vi "write_singleFIFO.vi"(10 "maximum bit depth":i8, 11 "values to be written":T1) -> (0 "FIFO overflow":bool)   [LabVIEW 2010]
uses:
  common_typedefs/channels_cluster.ctl
  <vilib>/rvi/DataTransferAndStorage/Container/XNode/niFpgaContainer.xnode
  <vilib>/rvi/DataTransferAndStorage/Container/Common/niFpgaContainerMethod.ctl
  <vilib>/rvi/DataTransferAndStorage/Container/Common/niFpgaTransferTypeControl.ctl
  <vilib>/rvi/interface/RandomDataEmulation/nirviRandomDataFPGAFIFO.vi
  <vilib>/rvi/interface/RandomDataEmulation/niFpgaRandomDataHandleErrors.vi
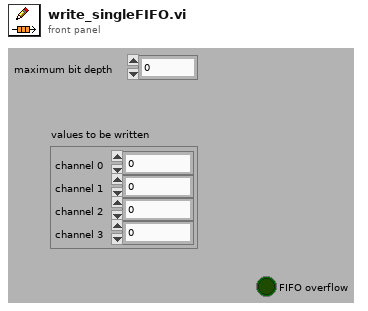
[diagram p1: front panel]
types:
  T1 = typedef "channels_cluster.ctl" = cluster{"channel 0":u32, "channel 1":u32, "channel 2":u32, "channel 3":u32}
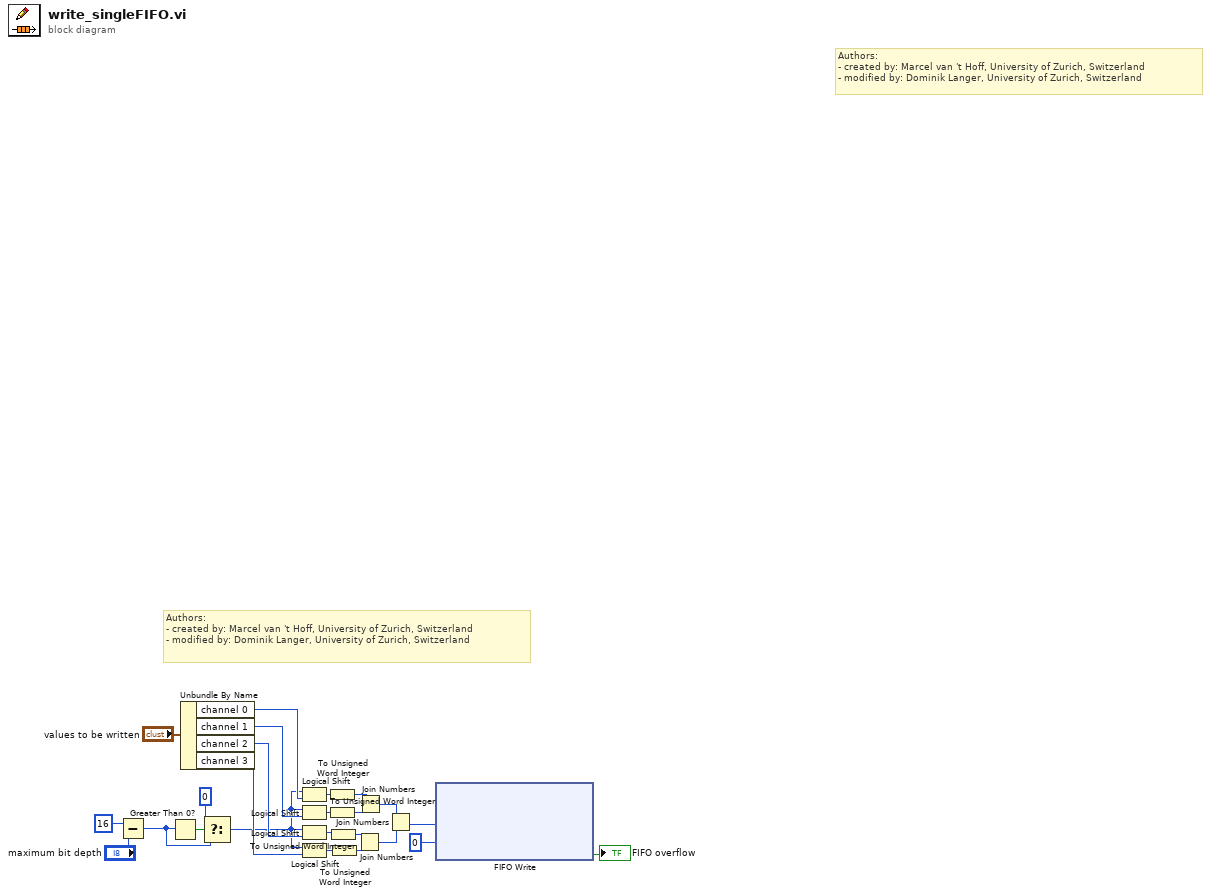
[diagram p0: block diagram]
diagram:
  # "Authors: \n- created by: Marcel van 't Hoff, University of Zurich, Switzerland\n- modified by: Dominik Langer, University of Zurich, Switzerland"
  # "Authors: \n- created by: Marcel van 't Hoff, University of Zurich, Switzerland\n- modified by: Dominik Langer, University of Zurich, Switzerland"
  n1 = Subtract(x=i8 16, y="maximum bit depth") -> (x-y=w20:i8)
  n2 = Greater Than 0?(x=w20) -> (x > 0?=w19:bool)
  n3 = Unbundle By Name("values to be written") -> ("channel 0"=w17:u32, "channel 1"=w18:u32, "channel 2"=w16:u32, "channel 3"=w13:u32)
  n4 = Select(t=i8 0 ("f"), s=w19, f=w20) -> (s? t:f=w12:i8)
  n5 = Logical Shift(y=w12, x=w17) -> (x << y=w8:u32)
  n6 = Logical Shift(y=w12, x=w18) -> (x << y=w6:u32)
  n7 = Logical Shift(y=w12, x=w16) -> (x << y=w3:u32)
  n8 = Logical Shift(y=w12, x=w13) -> (x << y=w5:u32)
  n9 = To Unsigned Word Integer(number=w8) -> (unsigned 16bit integer=w7:u16)
  n10 = To Unsigned Word Integer(number=w6) -> (unsigned 16bit integer=w1:u16)
  n11 = To Unsigned Word Integer(number=w3) -> (unsigned 16bit integer=w2:u16)
  n12 = To Unsigned Word Integer(number=w5) -> (unsigned 16bit integer=w4:u16)
  n13 = Join Numbers(hi=w2, lo=w4) -> ((hi.lo)=w10:u32)
  n14 = Join Numbers(hi=w7, lo=w1) -> ((hi.lo)=w11:u32)
  n15 = Join Numbers(hi=w11, lo=w10) -> ((hi.lo)=w9:u64)
  n16 = xnode ("FIFO Write")("Element"=w9, "Timeout"=0) -> ("Timed Out?"=→"FIFO overflow":bool)  [unwired: 1 in, 1 out]
